vi "Join-Data.vi"(0 "Existing Data":dbl[](array[numeric]), 2 "threshold":dbl=1.0, 11 "New Data":dbl[](array[numeric])) -> (8 "Output":dbl[](array[numeric]))   [LabVIEW 2011]
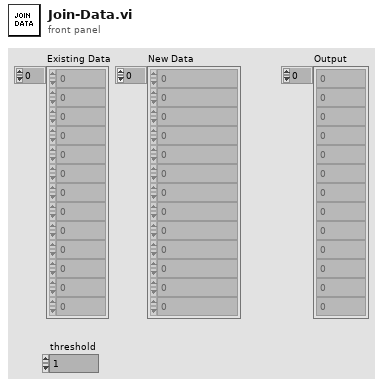
[diagram p1: front panel]
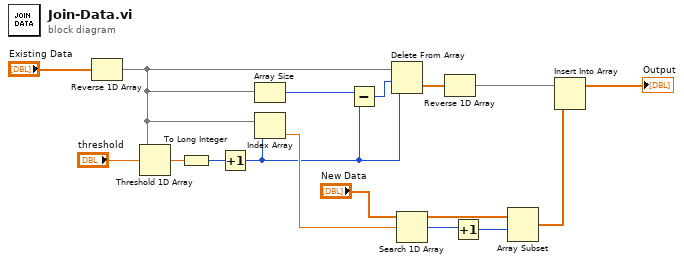
[diagram p0: block diagram]
diagram:
  n1 = Reverse 1D Array(array="Existing Data") -> (reversed array=w8:dbl[])
  n2 = Threshold 1D Array(2:"threshold", 3:w8) -> (0:w13:dbl)  [unwired: 1 in]
  n3 = To Long Integer(number=w13) -> (32bit integer=w10:i32)
  n4 = Increment(x=w10) -> (x+1=w7:i32)
  n5 = Array Size(array=w8) -> (size(s)=w9:i32)
  n6 = Index Array(array=w8, index=w7) -> (element=w14:dbl)
  n7 = Subtract(x=w9, y=w7) -> (x-y=w6:i32)
  n8 = Delete From Array(array=w8, length=w6, index=w7) -> (deleted portion=w5:dbl[])  [unwired: 1 out]
  n9 = Search 1D Array(1D array="New Data", element=w14) -> (index of element=w15:i32)  [unwired: 1 in]
  n10 = Reverse 1D Array(array=w5) -> (reversed array=w3:dbl[])
  n11 = Increment(x=w15) -> (x+1=w16:i32)
  n12 = Array Subset(array="New Data", index=w16) -> (w2:dbl[])  [unwired: 1 in]
  n13 = Insert Into Array(array=w3, new element=w2) -> (→"Output":dbl[])  [unwired: 1 in]
